vi "Phasor Convert Decay & Gates Parameters.vi"(11 "Phasor Parameters":T1={"Display Parameters"={"# Points"=0, "Ramp Type"=enum."Linear", "Type of Series"=enum."1-Exp Decays", "Min tau"=0.0, "Max tau"=0.0, "Include 0"=FALSE, "Include Infinity"=FALSE}, "Phasor Parameters"={"Harmonic Frequency"=0.0, "Use f* = 1/D Frequency"=FALSE, "Calibrated Phasor"=FALSE, "Calibration Lifetime"=1e-09, "Phasor Calculation"=enum."Direct Sum", "SEPL Type"=enum."UC", "# Gates"=1.0, "Square Gate Width"=1e-09, "Show Ticks"=FALSE}, "Decay & IRF Parameters"={"Lifetime"=0.0, "IRF Offset"=0.0, "IRF Period"=0.0, "Normalized Decays"=FALSE, "IRF Model"=enum."Dirac", "IRF Parameter 1"=0.0}, "Gate Parameters"={"First Gate Start"=0.0, "Use Gate Center"=FALSE, "Gate Width"=0.0, "Gate Step"=0.0, "# Gates"=0.0, "Gate Type"=enum."Square", "Edge Width"=0.0, "Top Slope"=0.0, "Reversed Sawtooth?"=FALSE, "Analytical Computation"=FALSE, "Integration"=enum."Item 0", "Tolerance"=1.0, "# Steps"=1.0, "Type of User-defined Function"=enum."Gate", "Use Gate Step"=FALSE}, "Detector Parameters"={"Frames/Image"=0, "Gates/Frame"=0, "Bits/Frame"=0, "Multiplicity"=0, "Incident Signal"=0.0, "Poisson Signal"=FALSE}} {"Detector Parameters"."Frames/Image" min=1; "Detector Parameters"."Multiplicity" min=0; "Detector Parameters"."Bits/Frame" min=1; "Detector Parameters"."Gates/Frame" min=1; "Gate Parameters"."# Steps" min=0.0; "Gate Parameters"."Tolerance" min=0.0; "Gate Parameters"."Top Slope" min=0.0; "Gate Parameters"."Edge Width" min=0.0; "Gate Parameters"."Gate Step" min=0.0; "Gate Parameters"."# Gates" min=0.0 step=1.0; "Gate Parameters"."Gate Width" min=0.0; "Decay & IRF Parameters"."Lifetime" min=0.0; "Decay & IRF Parameters"."IRF Period" min=0.0; "Phasor Parameters"."Square Gate Width" min=0.0; "Phasor Parameters"."# Gates" min=0.0; "Phasor Parameters"."Calibration Lifetime" min=0.0; "Phasor Parameters"."Harmonic Frequency" min=0.0; "Display Parameters"."Min tau" min=0.0; "Display Parameters"."Max tau" min=0.0; "Display Parameters"."# Points" min=1 step=1}) -> (2 "Gates Definitions":T14={"First Gate: t1"=0.0, "Gate Width: W"=0.0, "Gate Step: d"=0.0, "# Gates: G"=0.0, "Use Gate Center"=FALSE, "Frames/Image: F"=50, "Gates/Frame: L"=0, "Bits/Frame: q"=0, "Multiplicity: p"=0, "Gate Type"=enum."Square", "Gate Edge s"=4.0, "Gate Top Slope"=4.0, "Reversed Sawtooth?"=FALSE, "Computation"=FALSE, "User-defined Gate"={"X Array"=[], "Y Array"=[]}, "Tolerance"=50.0, "Integration"=enum."Item 0", "# Steps"=50.0, "Type of User-defined Function"=enum."Gate"}, 3 "Decay Definition":T13={"offset: t0"=0.0, "period: T"=0.0, "lifetime: tau"=0.0, "Incident Signal: I"=0.5, "Normalized Decays"=FALSE, "IRF Model"=enum."Dirac", "IRF Parameter 1"=0.0, "Poisson Signal"=FALSE})   [LabVIEW 2021, in "Phasor.lvlib"]
uses:
  Phasor.lvlib
  Phasor Gate Definitions.ctl
  Phasor Gate Type.ctl
  Graphs/XY Graph/XY Graph Plot Data.ctl
  Phasor Decay Definiton.ctl
  Phasor IRF Model.ctl
  Phasor SEPL Parameters.ctl
  Phasor Explorer Display Parameters.ctl
  Phasor Type of Series.ctl
  Phasor Explorer Phasor Parameters.ctl
  Phasor Calculation Type.ctl
  Phasor SEPL Type.ctl
  Phasor Explorer Decay Parameters.ctl
  Phasor Explorer Gate Parameters.ctl
  Phasor Type of User-defined Function.ctl
  Phasor Explorer Detector Parameters.ctl
  Phasor User-defined Gate & IRF.vi
  Graphs/XY Graph/XY Graph Add-Ons.lvlib
  Phasor Explorer.lvlib
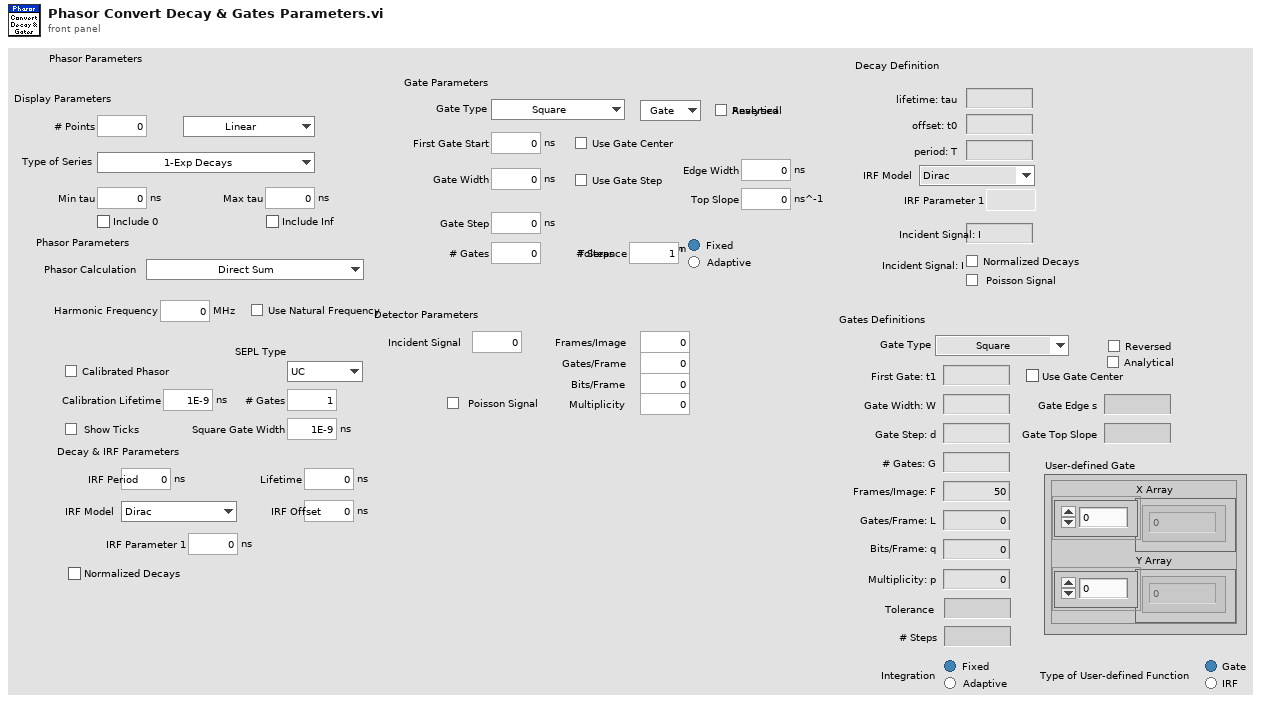
[diagram p1: front panel]
types:
  T1 = typedef "Phasor.lvlib/Phasor SEPL Parameters.ctl" = cluster{"Display Parameters":T2, "Phasor Parameters":T4, "Decay & IRF Parameters":T7, "Gate Parameters":T9, "Detector Parameters":T12}
  T2 = typedef "Phasor Explorer.lvlib/Phasor Explorer Display Parameters.ctl" = cluster{"# Points":i32, "Ramp Type":enum16{"Linear", "Logarithmic"}, "Type of Series":T3, "Min tau":dbl[unit], "Max tau":dbl[unit], "Include 0":bool, "Include Infinity":bool}
  T3 = typedef "Phasor.lvlib/Phasor Type of Series.ctl" = enum16{"1-Exp Decays", "Linear Combination of 1-Exp"}
  T4 = typedef "Phasor Explorer.lvlib/Phasor Explorer Phasor Parameters.ctl" = cluster{"Harmonic Frequency":dbl[unit], "Use f* = 1/D Frequency":bool, "Calibrated Phasor":bool, "Calibration Lifetime":dbl[unit], "Phasor Calculation":T5, "SEPL Type":T6, "# Gates":dbl, "Square Gate Width":dbl[unit], "Show Ticks":bool}
  T5 = typedef "Phasor.lvlib/Phasor Calculation Type.ctl" = enum16{"Direct Sum", "Analytical Formula"}
  T6 = typedef "Phasor.lvlib/Phasor SEPL Type.ctl" = enum16{"UC", "L_N", "L_N[W]", "L_X"}
  T7 = typedef "Phasor Explorer.lvlib/Phasor Explorer Decay Parameters.ctl" = cluster{"Lifetime":dbl[unit], "IRF Offset":dbl[unit], "IRF Period":dbl[unit], "Normalized Decays":bool, "IRF Model":T8, "IRF Parameter 1":dbl[unit]}
  T8 = typedef "Phasor.lvlib/Phasor IRF Model.ctl" = enum16{"Dirac", "Exponential"}
  T9 = typedef "Phasor Explorer.lvlib/Phasor Explorer Gate Parameters.ctl" = cluster{"First Gate Start":dbl[unit], "Use Gate Center":bool, "Gate Width":dbl[unit], "Gate Step":dbl[unit], "# Gates":dbl, "Gate Type":T10, "Edge Width":dbl[unit], "Top Slope":dbl[unit], "Reversed Sawtooth?":bool, "Analytical Computation":bool, "Integration":enum32{"Item 0", "Item 1"}, "Tolerance":dbl, "# Steps":dbl, "Type of User-defined Function":T11, "Use Gate Step":bool}
  T10 = typedef "Phasor.lvlib/Phasor Gate Type.ctl" = enum16{"Square", "Finite Edge Square", "Finite Edge, Tilted Top Square", "Triangle", "Sawtooth", "User-defined"}
  T11 = typedef "Phasor.lvlib/Phasor Type of User-defined Function.ctl" = enum16{"Gate", "IRF"}
  T12 = typedef "Phasor Explorer.lvlib/Phasor Explorer Detector Parameters.ctl" = cluster{"Frames/Image":i32, "Gates/Frame":i32, "Bits/Frame":i32, "Multiplicity":i32, "Incident Signal":dbl, "Poisson Signal":bool}
  T13 = typedef "Phasor.lvlib/Phasor Decay Definiton.ctl" = cluster{"offset: t0":ext, "period: T":ext, "lifetime: tau":ext, "Incident Signal: I":ext, "Normalized Decays":bool, "IRF Model":T8, "IRF Parameter 1":ext, "Poisson Signal":bool}
  T14 = typedef "Phasor.lvlib/Phasor Gate Definitions.ctl" = cluster{"First Gate: t1":ext, "Gate Width: W":ext, "Gate Step: d":ext, "# Gates: G":ext, "Use Gate Center":bool, "Frames/Image: F":i32, "Gates/Frame: L":i32, "Bits/Frame: q":i32, "Multiplicity: p":i32, "Gate Type":T10, "Gate Edge s":ext, "Gate Top Slope":ext, "Reversed Sawtooth?":bool, "Computation":bool, "User-defined Gate":T15, "Tolerance":ext, "Integration":enum32{"Item 0", "Item 1"}, "# Steps":ext, "Type of User-defined Function":enum32{"Gate", "IRF"}}
  T15 = typedef "XY Graph Add-Ons.lvlib/XY Graph Plot Data.ctl" = cluster{"X Array":dbl[], "Y Array":dbl[]}
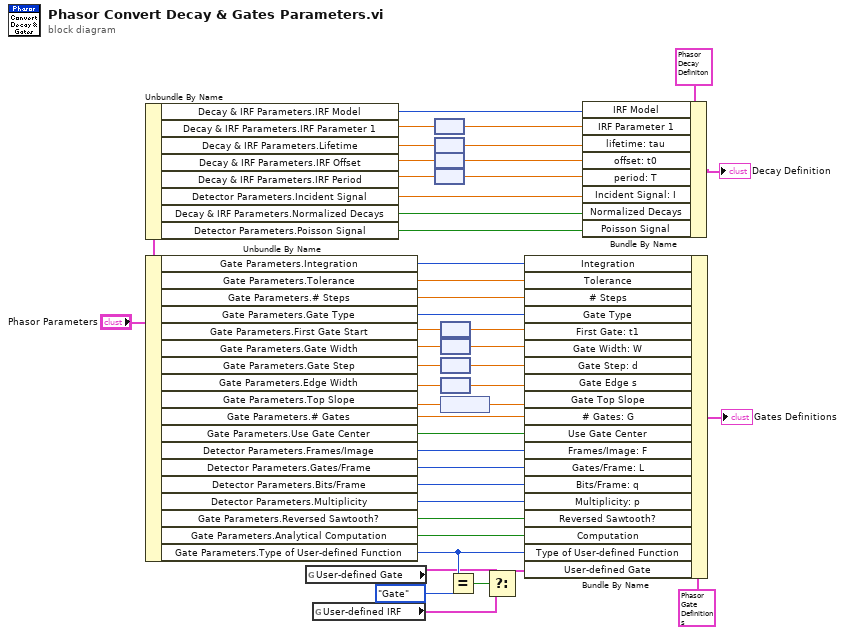
[diagram p0: block diagram]
diagram:
  n1 = Unbundle By Name("Phasor Parameters") -> ("Decay & IRF Parameters.IRF Model"=w14:T8, "Decay & IRF Parameters.IRF Parameter 1"=w13:dbl[unit], "Decay & IRF Parameters.Lifetime"=w22:dbl[unit], "Decay & IRF Parameters.IRF Offset"=w44:dbl[unit], "Decay & IRF Parameters.IRF Period"=w41:dbl[unit], "Detector Parameters.Incident Signal"=w34:dbl, "Decay & IRF Parameters.Normalized Decays"=w23:bool, "Detector Parameters.Poisson Signal"=w7:bool)
  n2 = Unbundle By Name("Phasor Parameters") -> ("Gate Parameters.Integration"=w9:enum32{"Item 0", "Item 1"}, "Gate Parameters.Tolerance"=w10:dbl, "Gate Parameters.# Steps"=w8:dbl, "Gate Parameters.Gate Type"=w21:T10, "Gate Parameters.First Gate Start"=w32:dbl[unit], "Gate Parameters.Gate Width"=w31:dbl[unit], "Gate Parameters.Gate Step"=w30:dbl[unit], "Gate Parameters.Edge Width"=w20:dbl[unit], "Gate Parameters.Top Slope"=w18:dbl[unit], "Gate Parameters.# Gates"=w29:dbl, "Gate Parameters.Use Gate Center"=w28:bool, "Detector Parameters.Frames/Image"=w27:i32, "Detector Parameters.Gates/Frame"=w26:i32, "Detector Parameters.Bits/Frame"=w25:i32, "Detector Parameters.Multiplicity"=w24:i32, "Gate Parameters.Reversed Sawtooth?"=w16:bool, "Gate Parameters.Analytical Computation"=w11:bool, "Gate Parameters.Type of User-defined Function"=w6:T11)
  n3 = global read "Phasor User-defined Gate & IRF.vi" "User-defined Gate"() -> (w2:T15)
  n4 = global read "Phasor User-defined Gate & IRF.vi" "User-defined IRF"() -> (w3:T15)
  n5 = node(w13) -> (w12:dbl)
  n6 = node(w22) -> (w42:dbl)
  n7 = node(w44) -> (w43:dbl)
  n8 = node(w41) -> (w40:dbl)
  n9 = node(w32) -> (w37:dbl)
  n10 = node(w31) -> (w36:dbl)
  n11 = node(w30) -> (w35:dbl)
  n12 = node(w20) -> (w19:dbl)
  n13 = node(w18) -> (w17:dbl)
  n14 = Equal?(x=w6, y=Phasor_Type_of_User-defined_Function."Gate") -> (x = y?=w4:bool)
  n15 = Select(t=w2, s=w4, f=w3) -> (s? t:f=w1:T15)
  n16 = Bundle By Name(cluster=T14 {"First Gate: t1"=0.0, "Gate Width: W"=4.0, "Gate Step: d"=0.3, "# Gates: G"=50.0, "Use Gate Center"=FALSE, "Frames/Image: F"=50, "Gates/Frame: L"=0, "Bits/Frame: q"=0, "Multiplicity: p"=0, "Gate Type"=enum."Square", "Gate Edge s"=4.0, "Gate Top Slope"=4.0, "Reversed Sawtooth?"=FALSE, "Computation"=FALSE, "User-defined Gate"={"X Array"=[], "Y Array"=[]}, "Tolerance"=50.0, "Integration"=enum."Item 0", "# Steps"=50.0, "Type of User-defined Function"=enum."Gate"} ("Gates Definitions"), "Integration"=w9, "Tolerance"=w10, "# Steps"=w8, "Gate Type"=w21, "First Gate: t1"=w37, "Gate Width: W"=w36, "Gate Step: d"=w35, "Gate Edge s"=w19, "Gate Top Slope"=w17, "# Gates: G"=w29, "Use Gate Center"=w28, "Frames/Image: F"=w27, "Gates/Frame: L"=w26, "Bits/Frame: q"=w25, "Multiplicity: p"=w24, "Reversed Sawtooth?"=w16, "Computation"=w11, "Type of User-defined Function"=w6, "User-defined Gate"=w1) -> (→"Gates Definitions":T14)
  n17 = Bundle By Name(cluster=T13 {"offset: t0"=2.0, "period: T"=15.0, "lifetime: tau"=0.5, "Incident Signal: I"=0.5, "Normalized Decays"=FALSE, "IRF Model"=enum."Dirac", "IRF Parameter 1"=0.0, "Poisson Signal"=FALSE} ("Decay Definition"), "IRF Model"=w14, "IRF Parameter 1"=w12, "lifetime: tau"=w42, "offset: t0"=w43, "period: T"=w40, "Incident Signal: I"=w34, "Normalized Decays"=w23, "Poisson Signal"=w7) -> (→"Decay Definition":T13)
